vi "dealer.vi"() -> ()   [LabVIEW 2012]
uses:
  <vilib>/addons/zeromq/socket_type.ctl
  <vilib>/addons/zeromq/socket_options.ctl
  <vilib>/addons/zeromq/zeromq.lvlib
panel:
  out "error out":errorcluster
  in  "endpoint":string="tcp://127.0.0.1:5557"
  out "Messages/Second(10 KiloBytes)":dbl
  out "Elapsed Seconds(10 KiloBytes)":dbl
  out "Messages/Second(1 KiloByte)":dbl
  out "Elapsed Seconds(1 KiloByte)":dbl
  out "Messages/Second(10 Bytes)":dbl
  out "Elapsed Seconds(10 Bytes)":dbl
  in  "Volume":i32=40000
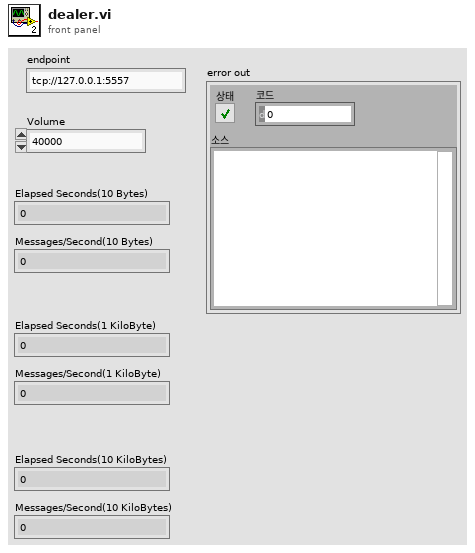
[diagram p1: front panel]
types:
  T1 = typedef "zeromq.lvlib/socket_options.ctl" = enum8{"NONE", "ZMQ_HWM", "<2>", "ZMQ_SWAP", "ZMQ_AFFINITY", "ZMQ_IDENTITY", "ZMQ_SUBSCRIBE", "ZMQ_UNSUBSCRIBE", "ZMQ_RATE", "ZMQ_RECOVERY_IVL", "ZMQ_MCAST_LOOP", "ZMQ_SNDBUF", "ZMQ_RCVBUF", "ZMQ_RCVMORE", "ZMQ_FD", "ZMQ_EVENTS", "ZMQ_TYPE", "ZMQ_LINGER", "ZMQ_RECONNECT_IVL", "ZMQ_BACKLOG", "ZMQ_RECOVERY_IVL_MSEC", "ZMQ_RECONNECT_IVL_MAX", "ZMQ_MAXMSGSIZE", "ZMQ_SNDHWM", "ZMQ_RCVHWM", "ZMQ_MULTICAST_HOPS", "<26>", "ZMQ_RCVTIMEO", "ZMQ_SNDTIMEO", "<29>", "<30>", "ZMQ_IPV4ONLY", "ZMQ_LAST_ENDPOINT", "ZMQ_ROUTER_MANDATORY", "ZMQ_TCP_KEEPALIVE", "ZMQ_TCP_KEEPALIVE_CNT", "ZMQ_TCP_KEEPALIVE_IDLE", "ZMQ_TCP_KEEPALIVE_INTVL", "ZMQ_TCP_ACCEPT_FILTER", "ZMQ_DELAY_ATTACH_ON_CONNECT", "ZMQ_XPUB_VERBOSE"}
  T2 = typedef "zeromq.lvlib/socket_type.ctl" = enum8{"ZMQ_PAIR", "ZMQ_PUB", "ZMQ_SUB", "ZMQ_REQ", "ZMQ_REP", "ZMQ_DEALER", "ZMQ_ROUTER", "ZMQ_PULL", "ZMQ_PUSH", "ZMQ_XPUB", "ZMQ_XSUB"}
  T3 = typedef "pointer.ctl" = u64
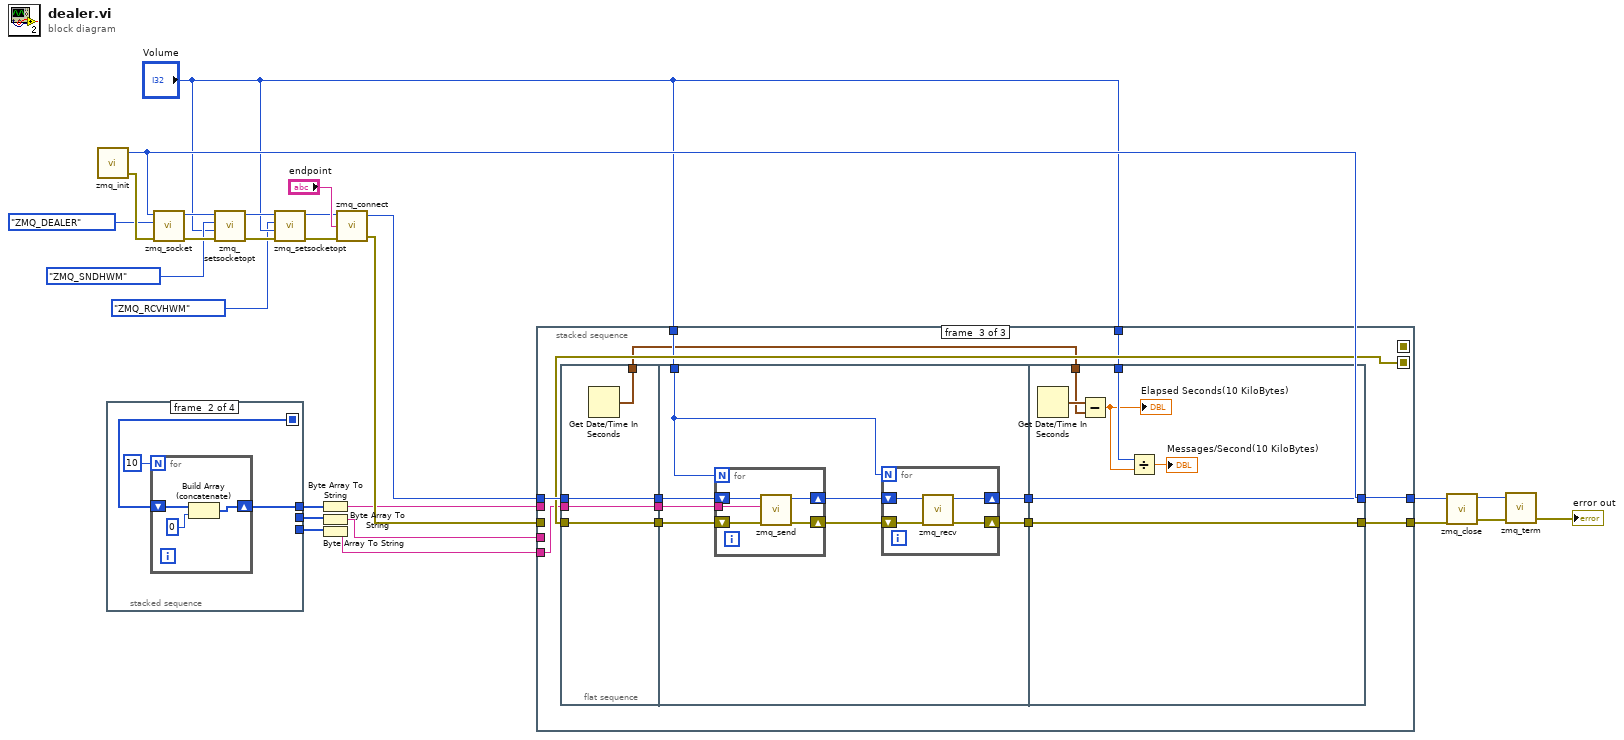
[diagram p0: block diagram]
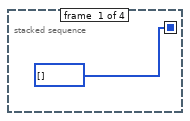
[diagram p2: hidden frame]
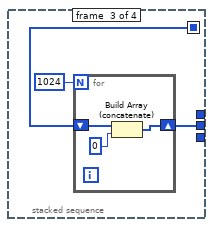
[diagram p3: hidden frame]
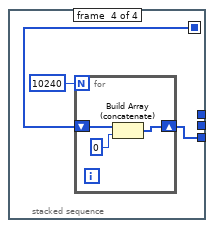
[diagram p4: hidden frame]
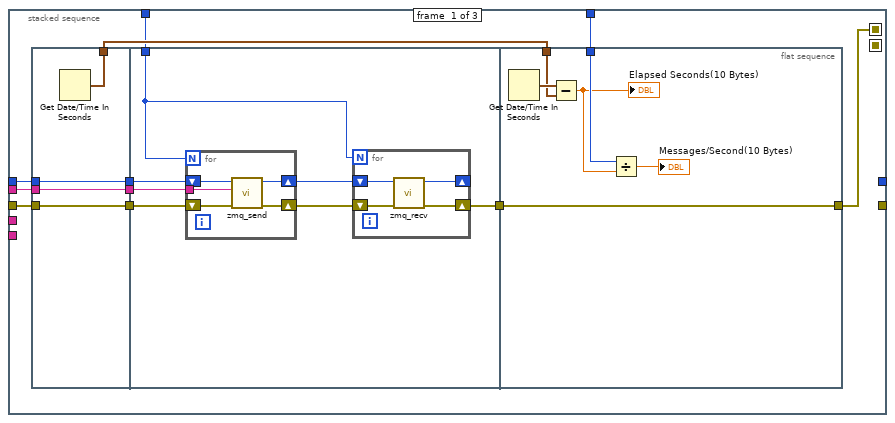
[diagram p5: hidden frame]
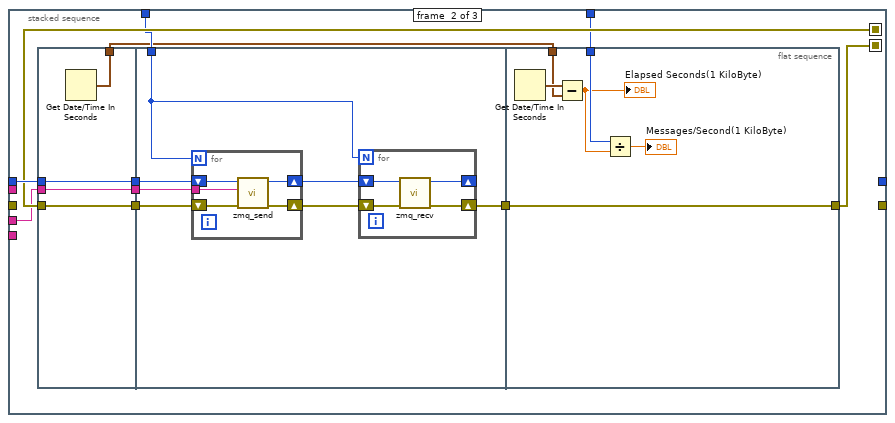
[diagram p6: hidden frame]
diagram:
  n1 = call <vilib>:"zmq_init.vi"() -> ("error out"=w25:errorcluster, "context"=w14:T3)  [unwired: 4 in]
  n2 = stacked-sequence {
    seq-local: [u8[] [] _ _ _] -> [_ w27 w33 w39]
    tunnel: [_ w28 _ _] -> w20
    tunnel: [_ _ w34 _] -> w18
    tunnel: [_ _ _ w40] -> w19
    frame #0 {
    }
    frame #1 {
      n3 = for {
        N: 10 -> [_]
        shift-right: [w30] -> w28
        shift-left: w27 -> [w32]
        n4 = Build Array (concatenate)(w32, u8 0 ("원소")) -> (w30:u8[])
      }
    }
    frame #2 {
      n5 = for {
        N: 1024 -> [_]
        shift-right: [w36] -> w34
        shift-left: w33 -> [w38]
        n6 = Build Array (concatenate)(w38, u8 0 ("원소")) -> (w36:u8[])
      }
    }
    frame #3 {
      n7 = for {
        N: 10240 -> [_]
        shift-right: [w42] -> w40
        shift-left: w39 -> [w44]
        n8 = Build Array (concatenate)(w44, u8 0 ("원소")) -> (w42:u8[])
      }
    }
  }
  n9 = call <vilib>:"zmq_socket.vi"("error in"=w25, "socket type"=socket_type."ZMQ_DEALER", "ctx in"=w14) -> ("error out"=w11:errorcluster, "socket"=w12:T3)  [unwired: 3 in]
  n10 = call <vilib>:"zmq_setsocketopt.vi"("error in"=w11, "value"="Volume", "option"=socket_options."ZMQ_SNDHWM", "socket in"=w12) -> ("error out"=w6:errorcluster, "socket out"=w9:T3)  [unwired: 2 in]
  n11 = call <vilib>:"zmq_setsocketopt.vi"("error in"=w6, "value"="Volume", "option"=socket_options."ZMQ_RCVHWM", "socket in"=w9) -> ("error out"=w7:errorcluster, "socket out"=w8:T3)  [unwired: 2 in]
  n12 = Byte Array To String(unsigned byte array=w20) -> (string=w3:string)
  n13 = Byte Array To String(unsigned byte array=w18) -> (string=w2:string)
  n14 = Byte Array To String(unsigned byte array=w19) -> (string=w1:string)
  n15 = call <vilib>:"zmq_connect.vi"("error in"=w7, "endpoint"="endpoint", "socket in"=w8) -> ("error out"=w22:errorcluster, "socket out"=w21:T3)  [unwired: 1 in]
  n16 = stacked-sequence {
    seq-local: [w46 _ _] -> [_ w87 _]
    seq-local: [_ w82 _] -> [_ _ w126]
    tunnel: "Volume" -> [w54 w86 w124]
    tunnel: w22 -> [w53 _ _]
    tunnel: w21 -> [w51 w88 w127]
    tunnel: w3 -> [w49 _ _]
    tunnel: "Volume" -> [w45 w83 w122]
    tunnel: w2 -> [_ w85 _]
    tunnel: w1 -> [_ _ w125]
    tunnel: [_ _ w121] -> w16
    tunnel: [_ _ w119] -> w17
    frame #0 {
      n17 = flat-sequence {
        tunnel: [w59] -> w55
        tunnel: w53 -> [w58]
        tunnel: [w58] -> w52
        tunnel: w51 -> [w57]
        tunnel: [w57] -> w50
        tunnel: w49 -> [w56]
        tunnel: [w56] -> w48
        tunnel: w54 -> [w63]
        tunnel: w52 -> [w66]
        tunnel: w50 -> [w65]
        tunnel: w48 -> [w64]
        tunnel: [w60] -> w47
        tunnel: w55 -> [w80]
        tunnel: w47 -> [w79]
        tunnel: [w79] -> w46
        tunnel: w45 -> [w77]
        frame #0 {
          n18 = Get Date/Time In Seconds() -> (seconds since 1Jan1904=w59:timestamp)
        }
        frame #1 {
          n19 = for {
            N: w63 -> [_]
            shift-right: [w71] -> w61
            shift-left: w66 -> [w74]
            shift-right: [w72] -> w62
            shift-left: w65 -> [w73]
            tunnel: w64 -> [w75]
            n20 = call <vilib>:"zmq_send.vi"("error in"=w74, "data"=w75, "socket in"=w73) -> ("error out"=w71:errorcluster, "socket out"=w72:T3)  [unwired: 4 in]
          }
          n21 = for {
            N: w63 -> [_]
            shift-right: [w67] -> _
            shift-left: w62 -> [w68]
            shift-right: [w69] -> w60
            shift-left: w61 -> [w70]
            n22 = call <vilib>:"zmq_recv.vi"("error in"=w70, "socket in"=w68) -> ("error out"=w69:errorcluster, "socket out"=w67:T3)  [unwired: 3 in, 3 out]
          }
        }
        frame #2 {
          n23 = Get Date/Time In Seconds() -> (seconds since 1Jan1904=w81:timestamp)
          n24 = Subtract(x=w81, y=w80) -> (x-y=w76:dbl)
          "Elapsed Seconds(10 Bytes)" <- w76
          n25 = Divide(x=w77, y=w76) -> (x/y=→"Messages/Second(10 Bytes)":dbl)
        }
      }
    }
    frame #1 {
      n26 = flat-sequence {
        tunnel: [w96] -> w84
        tunnel: w87 -> [w95]
        tunnel: [w95] -> w92
        tunnel: w88 -> [w94]
        tunnel: [w94] -> w91
        tunnel: w85 -> [w93]
        tunnel: [w93] -> w90
        tunnel: w86 -> [w100]
        tunnel: w92 -> [w103]
        tunnel: w91 -> [w102]
        tunnel: w90 -> [w101]
        tunnel: [w97] -> w89
        tunnel: w84 -> [w117]
        tunnel: w89 -> [w116]
        tunnel: [w116] -> w82
        tunnel: w83 -> [w114]
        frame #0 {
          n27 = Get Date/Time In Seconds() -> (seconds since 1Jan1904=w96:timestamp)
        }
        frame #1 {
          n28 = for {
            N: w100 -> [_]
            shift-right: [w108] -> w98
            shift-left: w103 -> [w111]
            shift-right: [w109] -> w99
            shift-left: w102 -> [w110]
            tunnel: w101 -> [w112]
            n29 = call <vilib>:"zmq_send.vi"("error in"=w111, "data"=w112, "socket in"=w110) -> ("error out"=w108:errorcluster, "socket out"=w109:T3)  [unwired: 4 in]
          }
          n30 = for {
            N: w100 -> [_]
            shift-right: [w104] -> _
            shift-left: w99 -> [w105]
            shift-right: [w106] -> w97
            shift-left: w98 -> [w107]
            n31 = call <vilib>:"zmq_recv.vi"("error in"=w107, "socket in"=w105) -> ("error out"=w106:errorcluster, "socket out"=w104:T3)  [unwired: 3 in, 3 out]
          }
        }
        frame #2 {
          n32 = Get Date/Time In Seconds() -> (seconds since 1Jan1904=w118:timestamp)
          n33 = Subtract(x=w118, y=w117) -> (x-y=w113:dbl)
          "Elapsed Seconds(1 KiloByte)" <- w113
          n34 = Divide(x=w114, y=w113) -> (x/y=→"Messages/Second(1 KiloByte)":dbl)
        }
      }
    }
    frame #2 {
      n35 = flat-sequence {
        tunnel: [w135] -> w123
        tunnel: w126 -> [w134]
        tunnel: [w134] -> w131
        tunnel: w127 -> [w133]
        tunnel: [w133] -> w130
        tunnel: w125 -> [w132]
        tunnel: [w132] -> w129
        tunnel: w124 -> [w140]
        tunnel: w131 -> [w143]
        tunnel: w130 -> [w142]
        tunnel: w129 -> [w141]
        tunnel: [w137] -> w128
        tunnel: [w136] -> w120
        tunnel: w123 -> [w158]
        tunnel: w128 -> [w157]
        tunnel: [w157] -> w121
        tunnel: w122 -> [w155]
        tunnel: w120 -> [w153]
        tunnel: [w153] -> w119
        frame #0 {
          n36 = Get Date/Time In Seconds() -> (seconds since 1Jan1904=w135:timestamp)
        }
        frame #1 {
          n37 = for {
            N: w140 -> [_]
            shift-right: [w148] -> w138
            shift-left: w143 -> [w151]
            shift-right: [w149] -> w139
            shift-left: w142 -> [w150]
            tunnel: w141 -> [w152]
            n38 = call <vilib>:"zmq_send.vi"("error in"=w151, "data"=w152, "socket in"=w150) -> ("error out"=w148:errorcluster, "socket out"=w149:T3)  [unwired: 4 in]
          }
          n39 = for {
            N: w140 -> [_]
            shift-right: [w144] -> w136
            shift-left: w139 -> [w145]
            shift-right: [w146] -> w137
            shift-left: w138 -> [w147]
            n40 = call <vilib>:"zmq_recv.vi"("error in"=w147, "socket in"=w145) -> ("error out"=w146:errorcluster, "socket out"=w144:T3)  [unwired: 3 in, 3 out]
          }
        }
        frame #2 {
          n41 = Get Date/Time In Seconds() -> (seconds since 1Jan1904=w159:timestamp)
          n42 = Subtract(x=w159, y=w158) -> (x-y=w154:dbl)
          "Elapsed Seconds(10 KiloBytes)" <- w154
          n43 = Divide(x=w155, y=w154) -> (x/y=→"Messages/Second(10 KiloBytes)":dbl)
        }
      }
    }
  }
  n44 = call <vilib>:"zmq_close.vi"("error in"=w16, "socket in"=w17) -> ("error out"=w15:errorcluster)  [unwired: 3 in]
  n45 = call <vilib>:"zmq_term.vi"("error in"=w15, "context"=w14) -> ("error out"=→"error out":errorcluster)  [unwired: 3 in]
